vi "Prompt_StartExp.vi"(5 "Project Strings":string[](array[string])=["UnspecifiedProj", "Proj_VaporTubes", "Proj_H2DT", "Proj_PIHVOF", "Proj_PIHVOF2", "Proj_SeedFeeder"], 6 "Measurement number":i32, 7 "Meas. Description":string="Init", 8 "SubFolder":string="Init", 9 "Project":u16(ring) items=["UnspecifiedProj", "Proj_VaporTubes", "Proj_H2DT", "Proj_PIHVOF", "Proj_PIHVOF2", "Proj_SeedFeeder"]) -> (0 "Experiment Description 2":string, 1 "Meas. Description 2":string="Init", 2 "SubFolder 2":string="Init", 3 "Project 2":u16(ring) items=["H2TC", "VAPOR1"], 4 "Measurement number 2":i32)   [LabVIEW 2018]
doc: "Displays a standard dialog box that prompts users to enter information, such as a user name and password.\n--------------------\n\nThis Express VI is configured as follows:\n\nMessage to Display to the User:\nThe inputs are: \nText Entry Box: Project\nText Entry Box: Measurement Description\nNumber: Measurement Number"
panel:
  in  "Experiment Description":string
  out "String 2":string="New Experiment" caption="String"
  out "error out":errorcluster
  in  "Enable":bool=TRUE
  in  "OK2":bool
  in  "OK1":bool
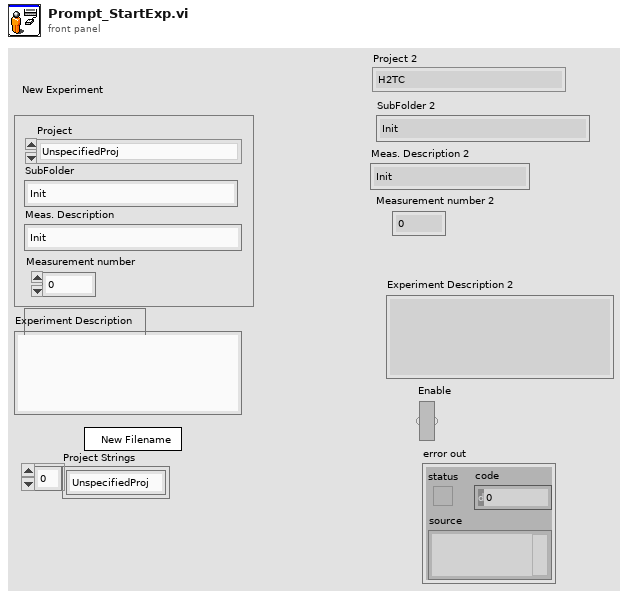
[diagram p1: front panel]
types:
  T1 = cluster{"Input Name":string, "Input Data Type":i32}[]
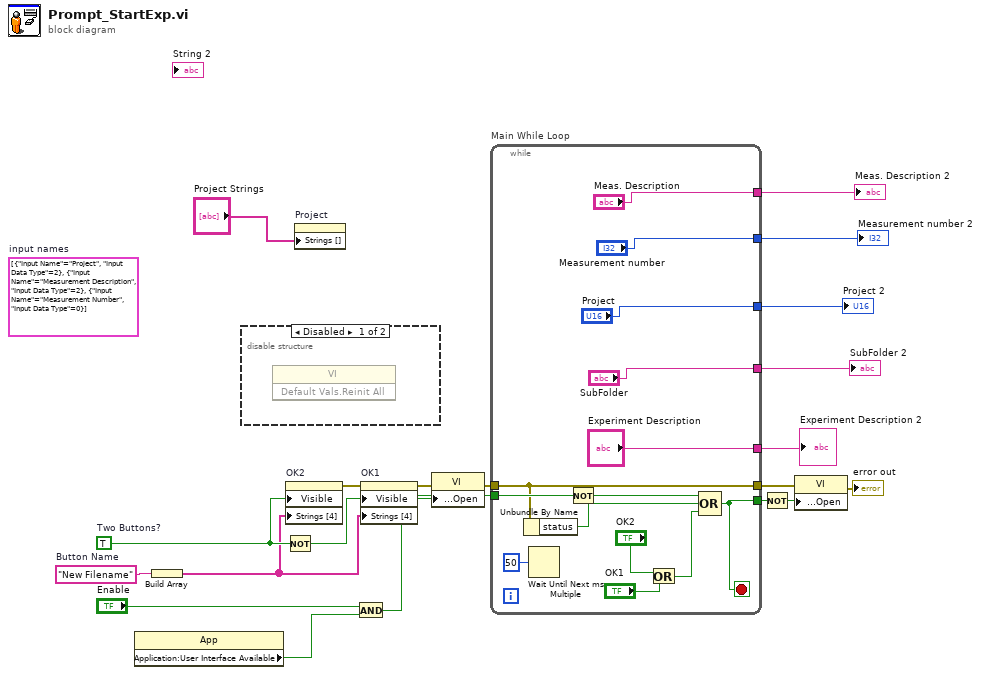
[diagram p0: block diagram]
diagram:
  (unwired) T1 [{"Input Name"="Project", "Input Data Type"=2}, {"Input Name"="Measurement Description", "Input Data Type"=2}, {"Input Name"="Measurement Number", "Input Data Type"=0}]  # input names
  w14 = "New Filename"  # Button Name
  w20 = TRUE  # Two Buttons?
  n1 = property class="App"() -> ("Application:User Interface Available"=w7:bool)  [unwired: 2 in, 2 out]
  n2 = Build Array(w14) -> (w15:string[])
  n3 = disable-structure shown="Disabled" {
    frame Disabled {
      n4 = invoke class="VI" method="Default Vals.Reinit All"() -> ()  [unwired: 3 in, 3 out]
    }
    frame Enabled {
    }
  }
  n5 = Not(x=w20) -> (.not. x?=w19:bool)
  n6 = property on="OK2" class="Bool"("Visible"=w20, "Strings [4]"=w15) -> (error out=w18:errorcluster)  [unwired: 2 in, 1 out]
  n7 = property on="Project" class="Ring (strict)"("Strings []"="Project Strings") -> ()  [unwired: 2 in, 2 out]
  n8 = And(x="Enable", y=w7) -> (x .and. y?=w8:bool)
  n9 = property on="OK1" class="Bool"(error in=w18, "Visible"=w19, "Strings [4]"=w15) -> (error out=w13:errorcluster)  [unwired: 1 in, 1 out]
  n10 = property class="VI"(error in=w13, "Front Panel Window:Open"=w8) -> (error out=w12:errorcluster)  [unwired: 1 in, 1 out]
  n11 = while "Main While Loop" {
    tunnel: w8 -> [w30]
    tunnel: [w28] -> w16
    tunnel: w12 -> [w27]
    tunnel: [w27] -> w11
    tunnel: ["Meas. Description"] -> w6
    tunnel: ["Measurement number"] -> w5
    tunnel: ["Project"] -> w4
    tunnel: ["SubFolder"] -> w3
    tunnel: ["Experiment Description"] -> w1
    stop <- w28 stop-if-true
    n12 = Unbundle By Name(w27) -> ("status"=w26:bool)
    n13 = Wait Until Next ms Multiple(millisecond multiple=u32 50) -> ()  [unwired: 1 out]
    n14 = Not(x=w30) -> (.not. x?=w29:bool)
    n15 = Or(x="OK2", y="OK1") -> (x .or. y?=w32:bool)
    n16 = Compound Arithmetic op=OR(w29, w26, w32) -> (w28:bool)
  }
  "Meas. Description 2" <- w6
  "Measurement number 2" <- w5
  "SubFolder 2" <- w3
  "Project 2" <- w4
  "Experiment Description 2" <- w1
  n17 = Not(x=w16) -> (.not. x?=w17:bool)
  n18 = property class="VI"(error in=w11, "Front Panel Window:Open"=w17) -> (error out=→"error out":errorcluster)  [unwired: 1 in, 1 out]
